vi "KneeSimControlPanel.vi"() -> ()   [LabVIEW 2026]
uses:
  <vilib>/Instr/_visa.llb/VISA Configure Serial Port (Instr).vi
panel:
  in  "Arduino Communication Port":refnum<visa-resource-name>
  out "Encoder Readings":T1
  in  "End Program":bool
  in  "Send Orientation":bool
  in  "ML Translation (mm)":dbl
  in  "AP Translation (mm)":dbl
  in  "VV Rotation (°)":dbl
  in  "IE Rotation (°)":dbl
  in  "FE Rotation (°)":dbl
  # "Flexion-Extension  (FE)  Boundaries: -20°,      160°\nInternal-External    (IE)   Boundaries: -65°,      65°\nVarus-Valgus          (VV) Boundaries: -10°,      10°\nAnterior-Posterior (AP) Boundaries: -20mm, 20mm\nMedial-Lateral       (ML) Boundaries: -20mm, 20mm"
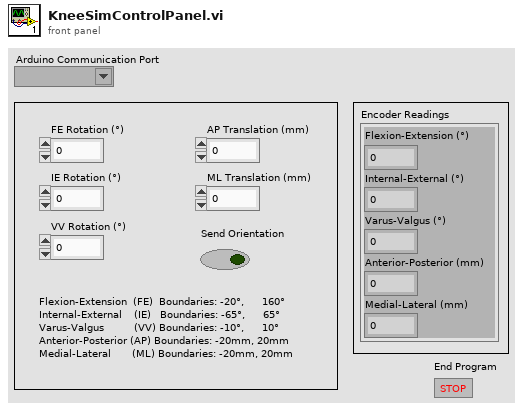
[diagram p1: front panel]
types:
  T1 = cluster{"Flexion-Extension (°)":dbl, "Internal-External (°)":dbl, "Varus-Valgus (°)":dbl, "Anterior-Posterior (mm)":dbl, "Medial-Lateral (mm)":dbl}
  T2 = cluster{"array type (2D Dbl)[0]":dbl, "array type (2D Dbl)[1]":dbl, "array type (2D Dbl)[2]":dbl, "array type (2D Dbl)[3]":dbl, "array type (2D Dbl)[4]":dbl}
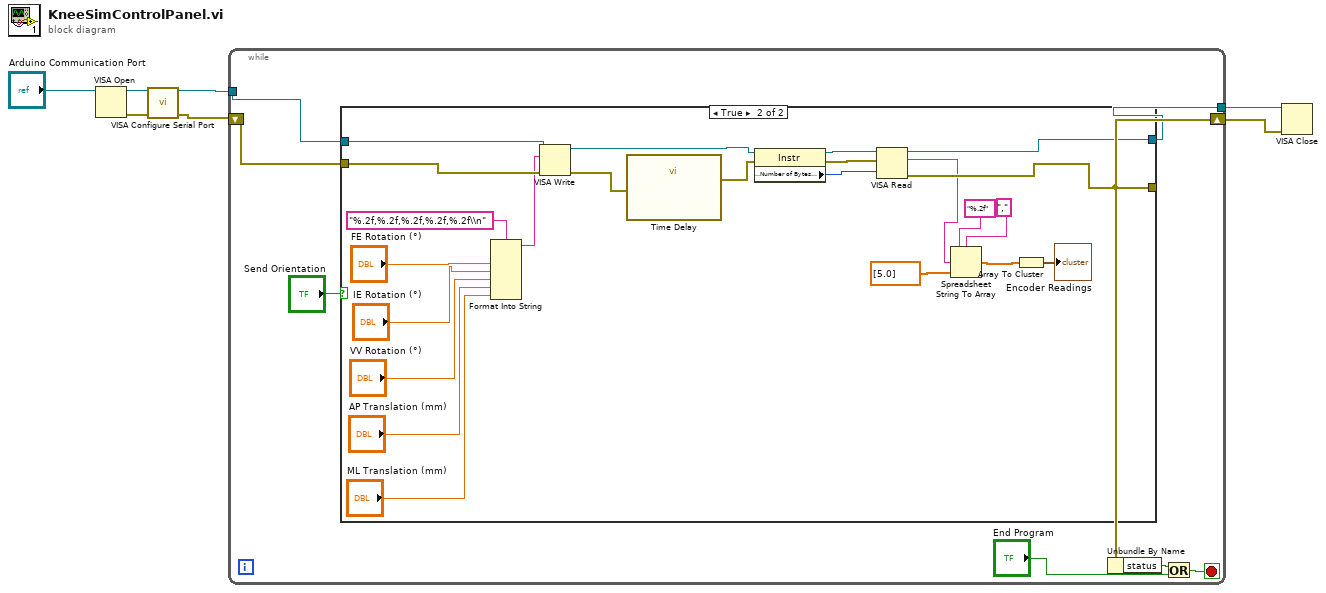
[diagram p0: block diagram]
diagram:
  n1 = VISA Open(VISA resource name="Arduino Communication Port") -> (VISA resource name=w6:refnum<visa-resource-name>, error out=w5:errorcluster)  [unwired: 4 in]
  n2 = call-poly "VISA Configure Serial Port"("VISA resource name"=w6, "error in (no error)"=w5) -> ("VISA resource name out"=w2:refnum<visa-resource-name>, "error out"=w4:errorcluster)  [unwired: 12 in]
  n3 = while {
    shift-right: [w13] -> w7
    shift-left: w4 -> [w15]
    tunnel: [w9] -> w3
    tunnel: w2 -> [w8]
    stop <- w14 stop-if-true
    n4 = case shown="True" "Send Orientation" {
      tunnel: w8 -> [w16 w39]
      tunnel: w15 -> [w17 w38]
      tunnel: [w16 w30] -> w9
      tunnel: [w17 w29] -> w13
      frame False {
      }
      frame True {
        n5 = Format Into String(format string="%.2f,%.2f,%.2f,%.2f,%.2f\\n", "FE Rotation (°)", "IE Rotation (°)", "VV Rotation (°)", "AP Translation (mm)", "ML Translation (mm)") -> (resulting string=w31:string)  [unwired: 2 in, 1 out]
        n6 = VISA Write(VISA resource name=w39, write buffer=w31, error in (no error)=w38) -> (VISA resource name out=w28:refnum<visa-resource-name>, error out=w40:errorcluster)  [unwired: 1 out]
        n7 = call "Time Delay"("error in (no error)"=w40) -> ("error out"=w27:errorcluster)  [unwired: 10 in]
        n8 = property class="Instr"(reference=w28, error in=w27) -> (reference out=w26:refnum<visa-resource-name>, error out=w25:errorcluster, "Serial Settings:Number of Bytes at Serial Port"=w24:u32)
        n9 = VISA Read(VISA resource name=w26, byte count=w24, error in (no error)=w25) -> (VISA resource name out=w30:refnum<visa-resource-name>, read buffer=w23:string, error out=w29:errorcluster)  [unwired: 1 out]
        n10 = Spreadsheet String To Array(delimiter (Tab)=",", format string="%.2f", spreadsheet string=w23, array type (2D Dbl)=dbl[] [5.0]) -> (array=w20:dbl[])
        n11 = Array To Cluster(array=w20) -> (cluster=→"Encoder Readings":T2)
      }
    }
    n12 = Unbundle By Name(w13) -> ("status"=w12:bool)
    n13 = Or(x=w12, y="End Program") -> (x .or. y?=w14:bool)
  }
  n14 = VISA Close(VISA resource name=w3, error in (no error)=w7) -> ()  [unwired: 1 out]
